vi "Create Framework Configuration.vi"(11 "Plugins":T4(array[cluster])=[{"plugin class"="udp", "channel count per transfer"=100, "transfer configs per group"=[], "group configs"=[], "plugin timing"={"priority"=0, "decimation"=1, "offset"=0}}]) -> (3 "Framework Configuration":T5)   [LabVIEW 2017]
uses:
  Source/Shared/Typedefs/DSF Framework Configuration.ctl
  Source/Shared/Typedefs/DSF Plugin Configuration.ctl
  Source/DSF Configuration API/1.0.0/Public/Controls/DSF Timing Info.ctl
  Source/Shared/Typedefs/DSF Transfer Group Configuration.ctl
  Source/DSF Configuration API/1.0.0/Public/Controls/DSF Direction.ctl
  Source/Shared/Typedefs/DSF Transfer Configuration.ctl
  Source/DSF Configuration API/1.0.0/Public/Controls/DSF Byte Order.ctl
  Source/Shared/Typedefs/DSF Channel Configuration.ctl
  Source/DSF Configuration API/1.0.0/Public/Controls/DSF Data Type.ctl
  Source/DSF Configuration API/1.0.0/Public/Controls/DSF Settings Info.ctl
  Source/DSF.Engine.lvlib
  Source/DSF Configuration API/1.0.0/DSF Configuration API.lvlib
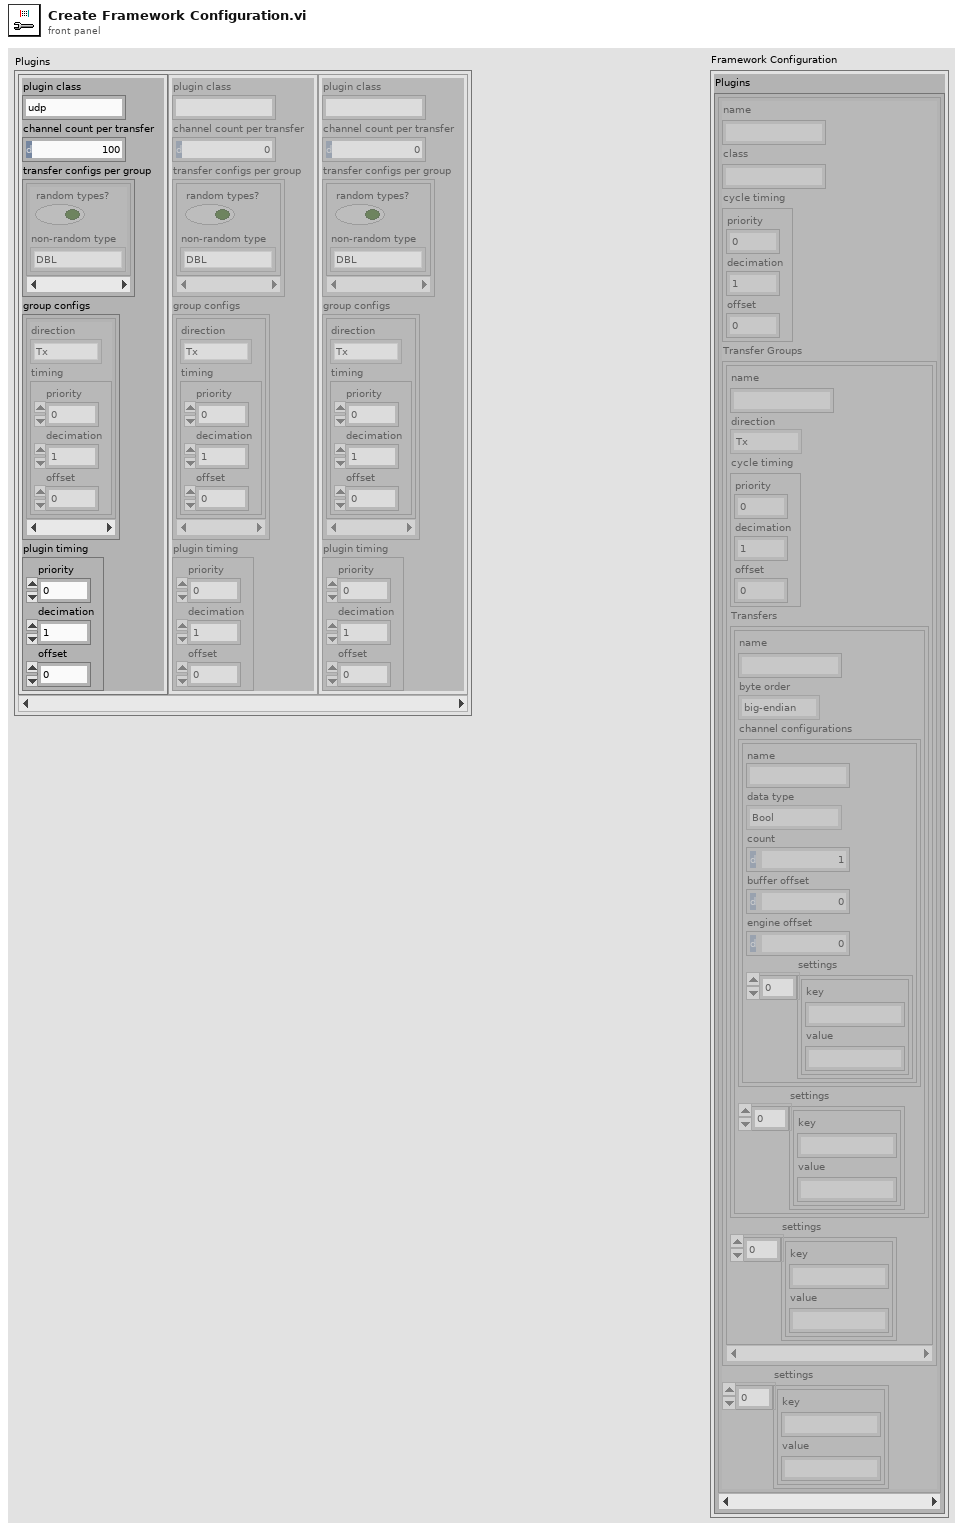
[diagram p1: front panel]
types:
  T1 = typedef "DSF Configuration API.lvlib/DSF Data Type.ctl" = enum8{"Bool", "SGL", "DBL", "I8", "I16", "I32", "I64", "U8", "U16", "U32", "U64"}
  T2 = typedef "DSF Configuration API.lvlib/DSF Direction.ctl" = enum8{"Tx", "Rx"}
  T3 = typedef "DSF Configuration API.lvlib/DSF Timing Info.ctl" = cluster{"priority":i32, "decimation":i32, "offset":i32}
  T4 = cluster{"plugin class":string, "channel count per transfer":i32, "transfer configs per group":cluster{"random types?":bool, "non-random type":T1}[], "group configs":cluster{"direction":T2, "timing":T3}[], "plugin timing":T3}[]
  T5 = typedef "DSF.Engine.lvlib/DSF Framework Configuration.ctl" = cluster{"Plugins":T6[]}
  T6 = typedef "DSF.Engine.lvlib/DSF Plugin Configuration.ctl" = cluster{"name":string, "class":string, "cycle timing":T3, "Transfer Groups":T7[], "settings":T11}
  T7 = typedef "DSF.Engine.lvlib/DSF Transfer Group Configuration.ctl" = cluster{"name":string, "direction":T2, "cycle timing":T3, "Transfers":T8[], "settings":T11}
  T8 = typedef "DSF.Engine.lvlib/DSF Transfer Configuration.ctl" = cluster{"name":string, "byte order":T9, "channel configurations":T10[], "settings":T11}
  T9 = typedef "DSF Configuration API.lvlib/DSF Byte Order.ctl" = enum8{"big-endian", "little-endian"}
  T10 = typedef "DSF.Engine.lvlib/DSF Channel Configuration.ctl" = cluster{"name":string, "data type":T1, "count":u64, "buffer offset":u64, "engine offset":u64, "settings":T11}
  T11 = typedef "DSF Configuration API.lvlib/DSF Settings Info.ctl" = cluster{"key":string, "value":string}[]
  T12 = cluster{"random types?":bool, "non-random type":T1}[]
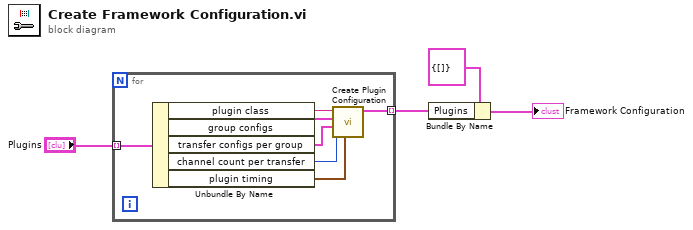
[diagram p0: block diagram]
diagram:
  n1 = for {
    tunnel: [w11] -> w3 mode=indexing
    tunnel: "Plugins" -> [w10] mode=indexing
    n2 = Unbundle By Name(w10) -> ("plugin class"=w9:string, "group configs"=w7:cluster{"direction":T2, "timing":T3}[], "transfer configs per group"=w5:T12, "channel count per transfer"=w6:i32, "plugin timing"=w8:T3)
    n3 = call "Create Plugin Configuration.vi"("plugin timing"=w8, "channel count per transfer"=w6, "transfer configs"=w5, "group configs"=w7, "plugin class"=w9) -> ("plugin configuration"=w11:T6)  [unwired: 6 in]
  }
  n4 = Bundle By Name(cluster=T5 {"Plugins"=[]} ("Framework Configuration"), "Plugins"=w3) -> (→"Framework Configuration":T5)
